vi "Main.vi"(11 "Module Admin":refnum<class "Delacor_lib_QMH_Module Admin.lvclass">) -> ()   [LabVIEW 2025, in "Power Supply.lvlib"]
doc: "This template is based from the Queued Message Handler design pattern and the Queued Message Handler Project Template that ships with LabVIEW 2014.\n\nThe main difference is that the Queue is private to this module and communication between modules is done via Broadcast and Request events.\n\nRequest events are wrapped via public API methods and are handled in the Event handler loop in this VI.\nAny module can register for Broadcast events sent by this module.\n\nThe Event Handling Loop generates messages based on user interface actions.\n\nThe Message Handling Loop processes messages generated by the Event Handling Loop, or by other messages. The messages are string values, so new messages can be added easily to the Message Cases case structure in the Message Handling Loop. Each message cluster can also provide an optional value for Message Data, which is a variant that can be converted to whatever message-specific data is required.\n_____\nBased on Delacor QMH Project Template 3.1.0.34.\n\n<b>Note:</b> This VI was modified by the <b>Validate DQMH Module</b> tool to add a call to the Error Reported VI at the end of the 'Exit' MHL frame.\n\n<b>Note:</b> This VI was modified by the <b>Validate DQMH Module</b> tool to call the Release Message Queue VI in the top-level Error case."
uses:
  Power Supply.lvlib
  <vilib>/Delacor/Delacor QMH/Libraries/Module Admin_class/Delacor_lib_QMH_Module Admin.lvclass
  <vilib>/MGI/Panel Manager/Panel/Panel/Panel.lvclass
  Module Data--cluster.ctl
  TV-STK-01/Plugins/PowerSupplies/PowerSupply/PowerSupply.lvlibp/PowerSupply/PowerSupply.lvclass
  Setpoints--cluster.ctl
  DC Output--enum.ctl
  Function Generator State--cluster.ctl
  Function Generator Parameters--cluster.ctl
  <vilib>/Utility/miscctls.llb/LVPointTypeDef.ctl
  <vilib>/Delacor/Delacor QMH/Libraries/Message Queue_class/Delacor_lib_QMH_Message Queue.lvclass/Delacor_lib_QMH_Message Queue.ctl
  Stop Argument--cluster.ctl
  <vilib>/Delacor/Delacor QMH/Libraries/Module Admin_class/Delacor_lib_QMH_Module Admin.lvclass/Delacor_lib_QMH_Module Admin.ctl
  Set Current SP Argument--cluster.ctl
  Set Voltage SP Argument--cluster.ctl
  Set Power SP Argument--cluster.ctl
  Set Power Supply Plugin Argument--cluster.ctl
  Set DC Output Argument--cluster.ctl
  Connect Argument--cluster.ctl
  Disconnect Argument--cluster.ctl
  Set Function Generator State Argument--cluster.ctl
  Set Function Generator Parameters Argument--cluster.ctl
  <vilib>/Delacor/Delacor QMH/Libraries/Message Queue_class/Delacor_lib_QMH_Enqueue Message (Single).vi
  <vilib>/Delacor/Delacor QMH/Libraries/Module Admin_class/Delacor_lib_QMH_Get External Launch.vi
  <vilib>/Utility/error.llb/Error Cluster From Error Code.vi
  <vilib>/ErrorRing/Error Ring.xnode
  <vilib>/Delacor/Delacor QMH/Libraries/Message Queue_class/Delacor_lib_QMH_Message Queue.lvclass
  <vilib>/MGI/Panel Manager/Panel/Panel Helper/Panel Helper.lvclass
  Get Status Argument--cluster.ctl
panel:
  out "Connected?":bool
  out "Function Generator State":T1
  out "Function Generator":T2
  out "Power Supply Status":T3
  out "Data Cluster":T4
  in  "Panel":refnum<class "Panel.lvclass">
  in  "Simulate MHL Error":bool
  in  "Simulate EHL Error":bool
  out "error out":errorcluster
  out "Status":string
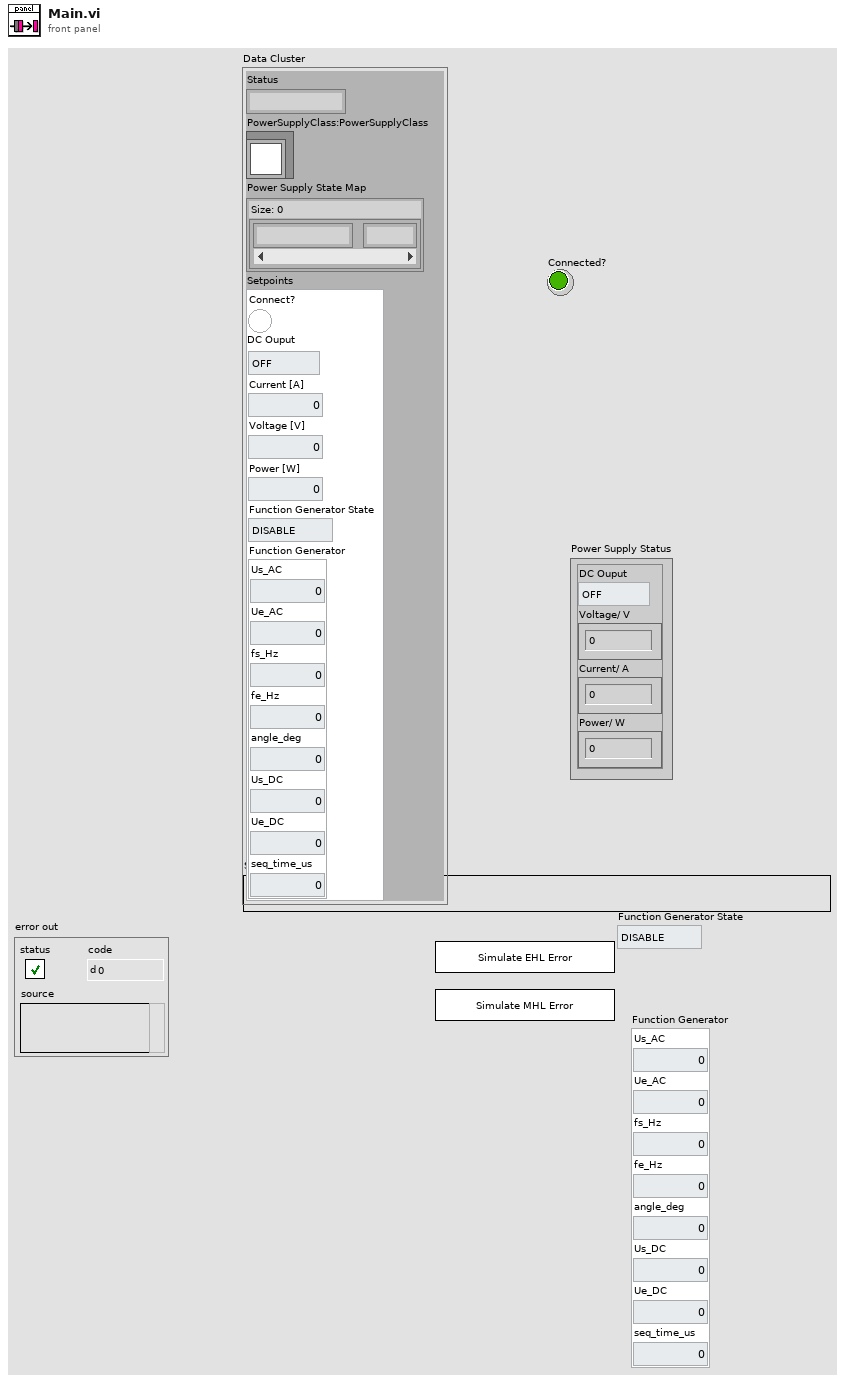
[diagram p1: front panel]
types:
  T1 = typedef "Power Supply.lvlib/Function Generator State--cluster.ctl" = enum16{"DISABLE", "ENABLE"}
  T2 = typedef "Power Supply.lvlib/Function Generator Parameters--cluster.ctl" = cluster{"Us_AC":sgl, "Ue_AC":sgl, "fs_Hz":sgl, "fe_Hz ":sgl, "angle_deg ":sgl, "Us_DC ":sgl, "Ue_DC":sgl, "seq_time_us":sgl}
  T3 = cluster{"DC Ouput":enum16{"OFF", "ON"}, "Voltage/ V":dbl, "Current/ A":dbl, "Power/ W":dbl}
  T4 = typedef "Power Supply.lvlib/Module Data--cluster.ctl" = cluster{"Status":string, "PowerSupplyClass:PowerSupplyClass":refnum<class "PowerSupply.lvclass">, "Power Supply State Map":map{string, dbl}, "Setpoints":T5}
  T5 = typedef "Power Supply.lvlib/Setpoints--cluster.ctl" = cluster{"Connect?":bool, "DC Ouput":T6, "Current [A]":dbl, "Voltage [V]":dbl, "Power [W]":dbl, "Function Generator State":T1, "Function Generator":T2}
  T6 = typedef "Power Supply.lvlib/DC Output--enum.ctl" = enum16{"OFF", "ON"}
  T7 = typedef "LVPointTypeDef.ctl" = cluster{"Horizontal":i16, "Vertical":i16}
  T8 = typedef "Power Supply.lvlib/Request Events--cluster.ctl" = cluster{"Stop Module":refnum<user-event>, "Show Panel":refnum<user-event>, "Hide Panel":refnum<user-event>, "Get Module Execution Status":refnum<user-event>, "Show Diagram":refnum<user-event>, "Change Panel":refnum<user-event>, "Set Current SP":refnum<user-event>, "Set Voltage SP":refnum<user-event>, "Set Power SP":refnum<user-event>, "Set Power Supply Plugin":refnum<user-event>, "Set DC Output":refnum<user-event>, "Private":cluster{"Sleep Connection Helper Loop":refnum<user-event>}, "Connect":refnum<user-event>, "Disconnect":refnum<user-event>, "Set Function Generator State":refnum<user-event>, "Private.Wake Connection Helper Loop":refnum<user-event>, "Private.Set DC Current SP":refnum<user-event>, "Private.Set DC Voltage SP":refnum<user-event>, "Private.Set DC Power SP":refnum<user-event>, "Private.Set DC Output SP":refnum<user-event>, "Set Function Generator Parameters":refnum<user-event>, "Private.Set Function Generator Parameters SP":refnum<user-event>, "Private.Set Function Generator State SP":refnum<user-event>}
  T9 = typedef "Panel.lvlib/Panel Helper.lvclass/Panel Events.ctl" = cluster{"My Panel":refnum<user-event>, "Top Level Initialized":refnum<user-event>}
  T10 = typedef "Power Supply.lvlib/Get Status Argument--cluster.ctl" = cluster{"Boolean":bool}
  T11 = typedef "Power Supply.lvlib/Stop Argument--cluster.ctl" = cluster{"Origin":string, "Exit via Stop Module Req?":bool, "Wait for Module to stop?":bool}
  T12 = typedef "Power Supply.lvlib/Set Current SP Argument--cluster.ctl" = cluster{"Current SP [A]":dbl}
  T13 = typedef "Power Supply.lvlib/Set Voltage SP Argument--cluster.ctl" = cluster{"Voltage SP [V]":dbl}
  T14 = typedef "Power Supply.lvlib/Set Power SP Argument--cluster.ctl" = cluster{"Power [W]":dbl}
  T15 = typedef "Power Supply.lvlib/Set Power Supply Plugin Argument--cluster.ctl" = cluster{"Plugin File Path":path}
  T16 = typedef "Power Supply.lvlib/Set DC Output Argument--cluster.ctl" = cluster{"DC Ouput":T6}
  T17 = typedef "Power Supply.lvlib/Connect Argument--cluster.ctl" = cluster{"Boolean":bool}
  T18 = typedef "Power Supply.lvlib/Disconnect Argument--cluster.ctl" = cluster{"Boolean":bool}
  T19 = typedef "Power Supply.lvlib/Set Function Generator State Argument--cluster.ctl" = cluster{"Function Generator State":T1}
  T20 = typedef "Power Supply.lvlib/Set Function Generator Parameters Argument--cluster.ctl" = cluster{"Function Generator":T2}
  T21 = enum32{"invalid lock state", "Not Locked", "Locked (No Password)", "Password-protected"}
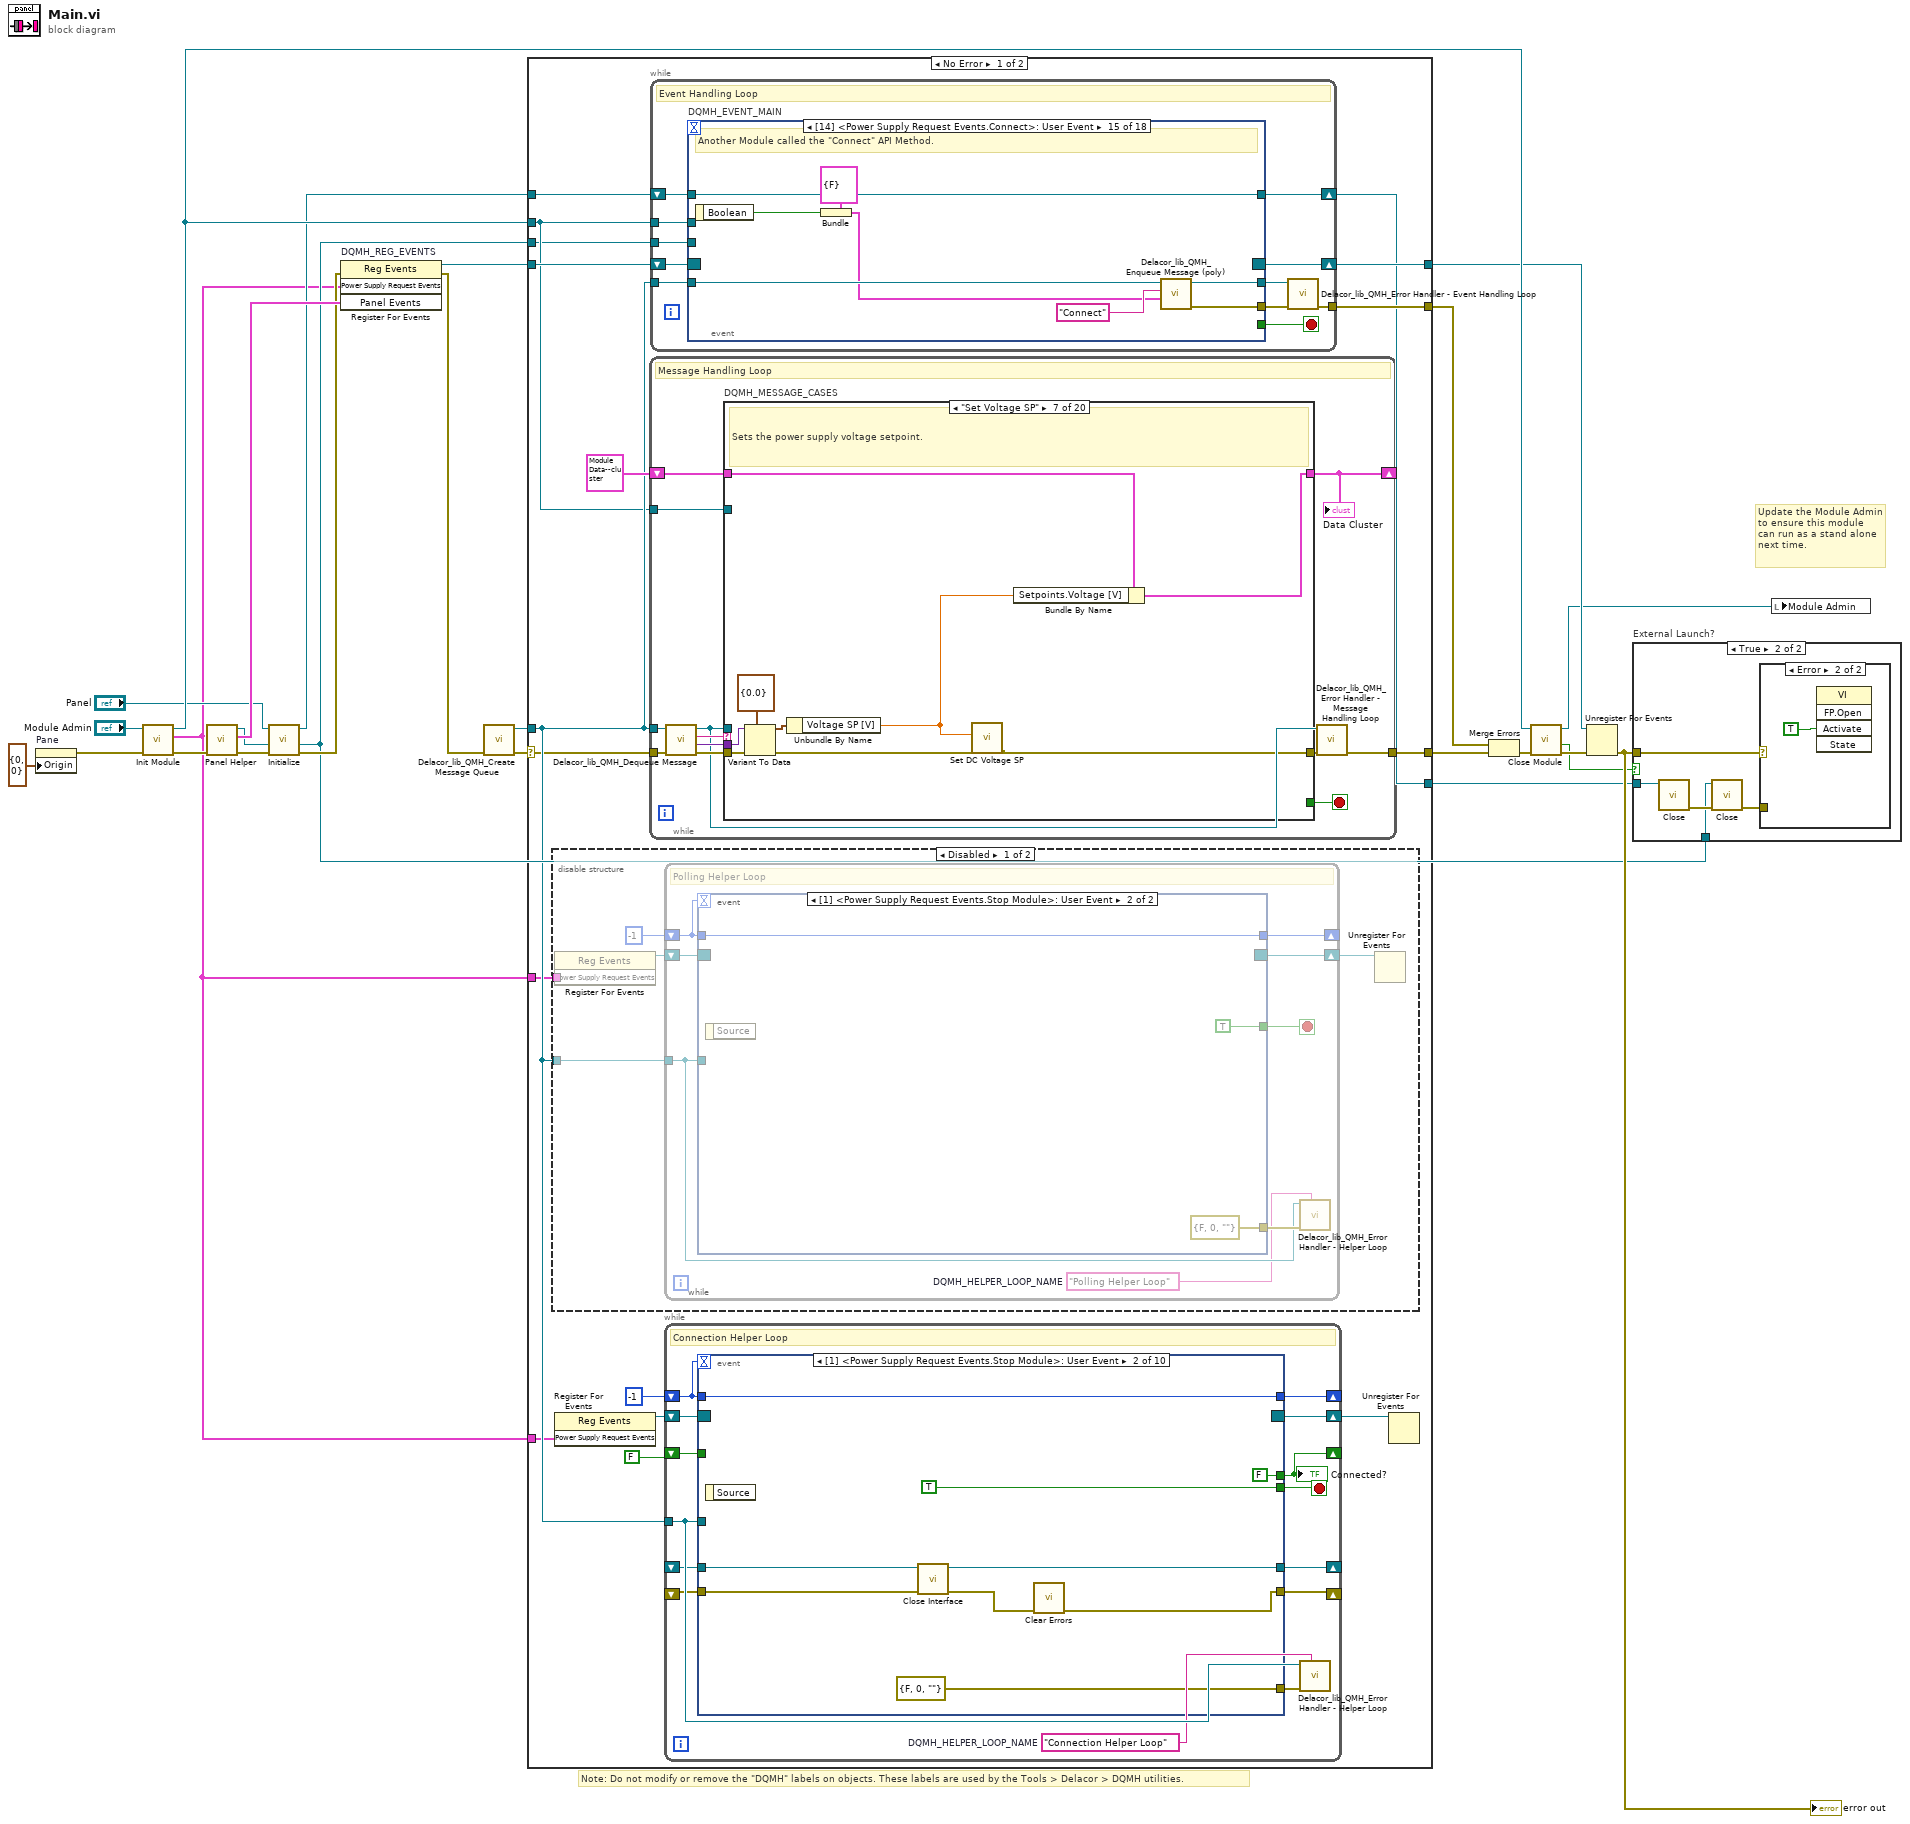
[diagram p0: block diagram]
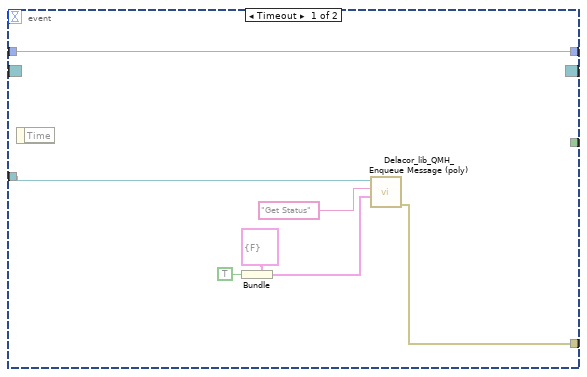
[diagram p4: hidden frame]
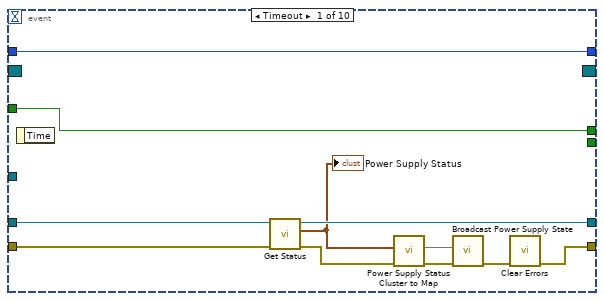
[diagram p6: hidden frame]
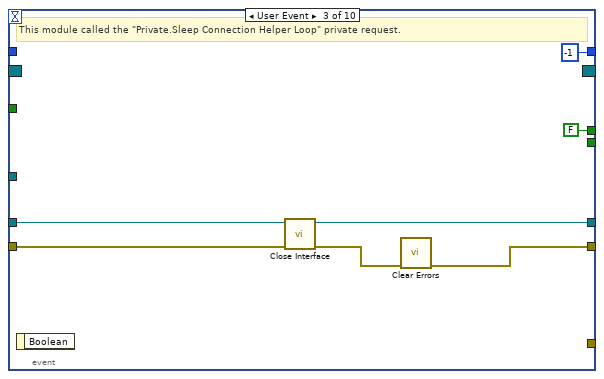
[diagram p7: hidden frame]
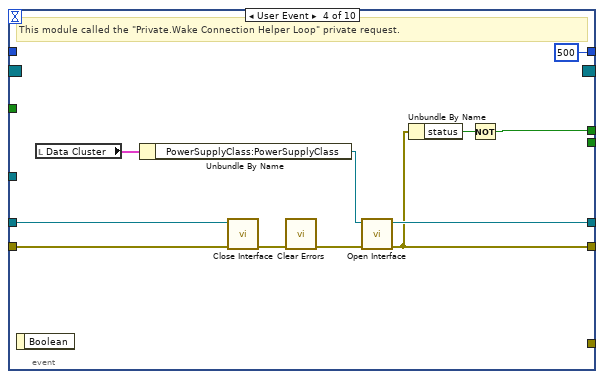
[diagram p8: hidden frame]
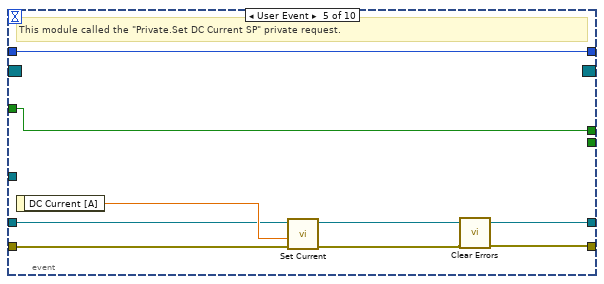
[diagram p9: hidden frame]
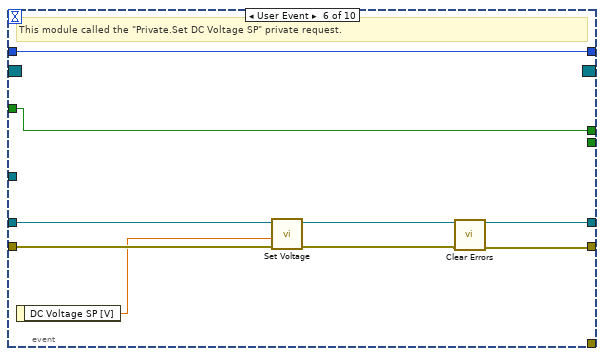
[diagram p10: hidden frame]
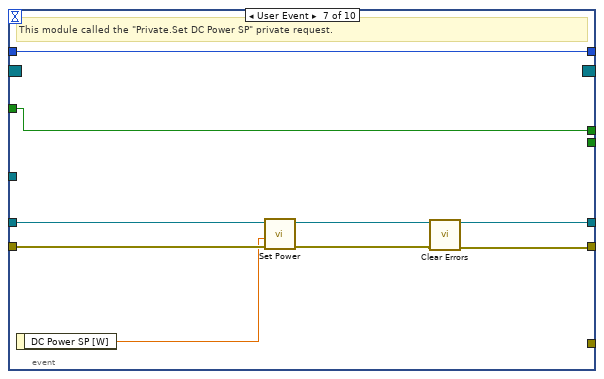
[diagram p11: hidden frame]
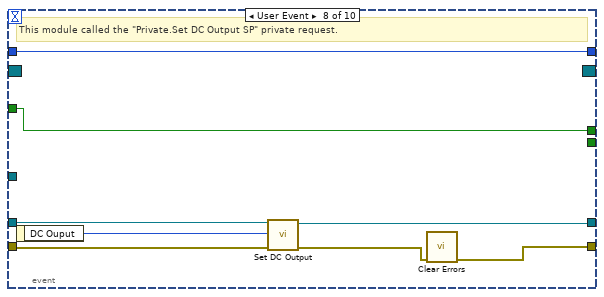
[diagram p12: hidden frame]
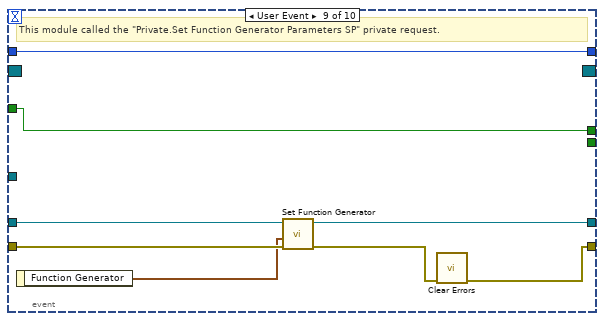
[diagram p13: hidden frame]
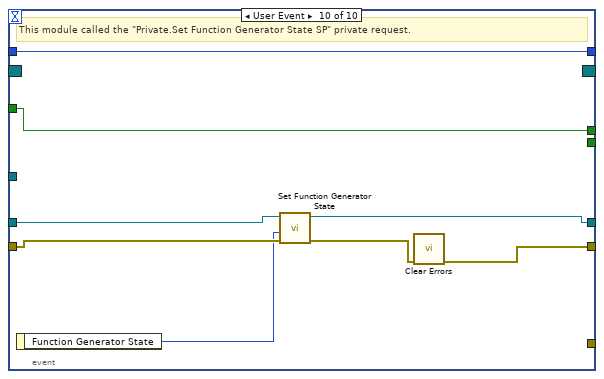
[diagram p14: hidden frame]
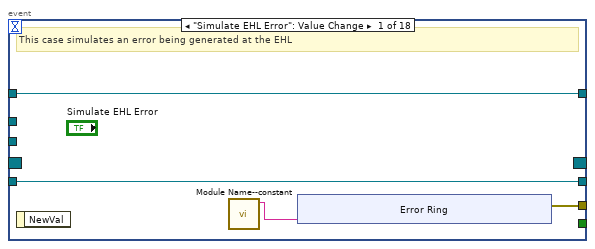
[diagram p15: hidden frame]
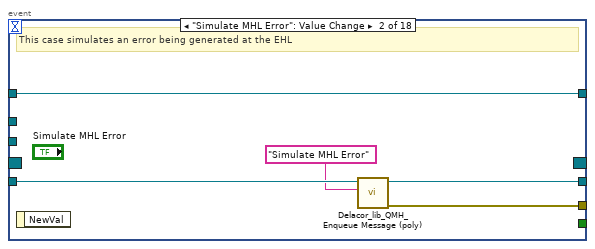
[diagram p16: hidden frame]
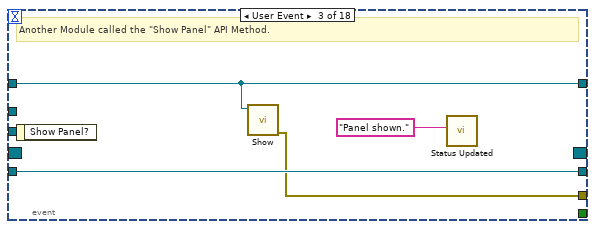
[diagram p17: hidden frame]
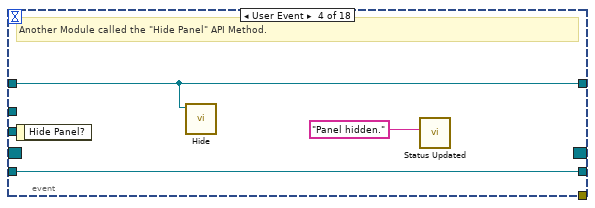
[diagram p18: hidden frame]
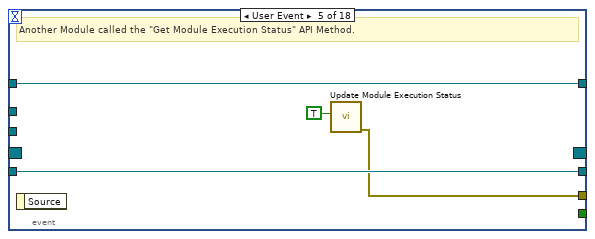
[diagram p19: hidden frame]
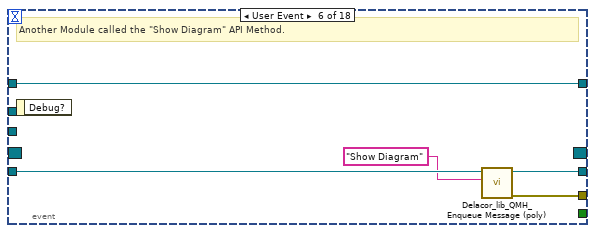
[diagram p20: hidden frame]
diagram:
  # "Note: Do not modify or remove the \"DQMH\" labels on objects. These labels are used by the Tools > Delacor > DQMH utilities."
  # "Update the Module Admin to ensure this module can run as a stand alone next time."
  n1 = property on="Pane" class="Pane"("Origin"=T7 {"Horizontal"=0, "Vertical"=0}) -> (error out=w2:errorcluster)  [unwired: 2 in, 1 out]
  n2 = call "Init Module.vi"("error in (no error)"=w2, "Singleton Module Admin in"="Module Admin") -> ("error out"=w12:errorcluster, "Power Supply Request Events"=w1:T8, "Singleton Module Admin out"=w26:refnum<class "Delacor_lib_QMH_Module Admin.lvclass">)  [unwired: 7 in]
  n3 = call <vilib>:"Panel Helper.vi"("Error In"=w12) -> ("Error Out"=w9:errorcluster, "Panel Events"=w11:T9, "Panel Helper out"=w8:refnum<class "Panel Helper.lvclass">)  [unwired: 8 in]
  n4 = call <vilib>:"Initialize.vi"("error in (no error)"=w9, "My Helper in"=w8, "Panel In"="Panel") -> ("error out"=w6:errorcluster, "My Helper out"=w5:refnum<class "Panel Helper.lvclass">, "Panel Out"=w4:refnum<class "Panel.lvclass">)  [unwired: 6 in]
  n5 = register-events "DQMH_REG_EVENTS"(error in=w6, w1, w11) -> (reference out=w23:refnum<event-registration>, error out=w10:errorcluster)  [unwired: 1 in]
  n6 = call <vilib>:"Delacor_lib_QMH_Create Message Queue.vi"("error in"=w10) -> ("error out"=w14:errorcluster, "Message Queue"=w22:refnum<class "Delacor_lib_QMH_Message Queue.lvclass">)  [unwired: 9 in]
  n7 = case shown="No Error" w14 {
    selector: w14 -> [w37 w520]
    tunnel: [w43 w520] -> w25
    tunnel: [w42 w525] -> w24
    tunnel: w23 -> [w40 w525]
    tunnel: w22 -> [w39 w516]
    tunnel: [w38 _] -> w18
    tunnel: w26 -> [w36 w521]
    tunnel: w4 -> [w34 w517]
    tunnel: w5 -> [w35 _]
    tunnel: [w33 w517] -> w13
    tunnel: w1 -> [w32 _]
    tunnel: w1 -> [w31 _]
    frame No Error {
      n8 = disable-structure shown="Disabled" {
        disable-tunnel: w39 -> [w48 _]
        disable-tunnel: w32 -> [w47 _]
        frame Disabled {
          n9 = register-events ("DQMH_HELPER_REGFOREVENTS")(w47) -> (reference out=w45:refnum<event-registration>)  [unwired: 2 in, 1 out]
          n10 = while "DQMH_HELPER_LOOP" {
            shift-right: [w56] -> _
            shift-left: -1 -> [w55]
            shift-right: [w53] -> w46
            shift-left: w45 -> [w54]
            tunnel: w48 -> [w50]
            stop <- w52 stop-if-true
            w49 = "Polling Helper Loop"  # DQMH_HELPER_LOOP_NAME
            # "Polling Helper Loop"
            n11 = event "DQMH_HELPER_EVENT_STRUCTURE" shown="[1] <Power Supply Request Events.Stop Module>: User Event" {
              selector: w54 -> [_ _]
              dyn-events: [_ _] -> w53
              timeout: w55 -> [_ _]
              tunnel: w55 -> [w63 w66]
              tunnel: [w63 w66] -> w56
              tunnel: [_ TRUE] -> w52
              tunnel: [w62 errorcluster {"status"=FALSE, "code"=0, "source"=""} ("error constant")] -> w51
              tunnel: w50 -> [w57 _]
              event Timeout {
                n12 = event-data() -> ()  [unwired: 1 in, 1 out]
                n13 = Bundle(cluster=T10 {"Boolean"=FALSE} ("Get Status Argument"), "Boolean"=TRUE) -> (w59:T10)
                n14 = call-poly <vilib>:"Delacor_lib_QMH_Enqueue Message (poly).vi"("Message Data"=w59, "Message"="Get Status", "Message Queue in"=w57) -> ("error out"=w62:errorcluster)  [unwired: 7 in, 1 out]
              }
              event User Event {
                n15 = event-data() -> ()  [unwired: 1 in, 1 out]
              }
            }
            n16 = call-dynamic "Delacor_lib_QMH_Error Handler - Helper Loop.vi"("Error Debug"=w49, "error in"=w51, "Message Queue in"=w50) -> ()  [unwired: 7 in, 2 out]
          }
          n17 = Unregister For Events(event registration refnum=w46) -> ()  [unwired: 1 in, 1 out]
        }
        frame Enabled {
        }
      }
      n18 = register-events ("DQMH_HELPER_REGFOREVENTS")(w31) -> (reference out=w29:refnum<event-registration>)  [unwired: 2 in, 1 out]
      n19 = while {
        tunnel: w39 -> [w323]
        shift-right: [w329] -> _
        shift-left: T4 {"Status"="", "PowerSupplyClass:PowerSupplyClass"=refnum, "Power Supply State Map"={}, "Setpoints"={"Connect?"=FALSE, "DC Ouput"=enum."OFF", "Current [A]"=0.0, "Voltage [V]"=0.0, "Power [W]"=0.0, "Function Generator State"=enum."DISABLE", "Function Generator"={"Us_AC"=0.0, "Ue_AC"=0.0, "fs_Hz"=0.0, "fe_Hz "=0.0, "angle_deg "=0.0, "Us_DC "=0.0, "Ue_DC"=0.0, "seq_time_us"=0.0}}} ("Data Cluster") -> [w330]
        tunnel: w37 -> [w327]
        tunnel: [w321] -> w43
        tunnel: w36 -> [w320]
        stop <- w328 stop-if-true
        # "Message Handling Loop"
        n20 = call-dynamic "Delacor_lib_QMH_Dequeue Message.vi"("error in"=w327, "Message Queue in"=w323) -> ("error out"=w326:errorcluster, "Message Data"=w324:variant, "Message"=w325:string, "Message Queue out"=w322:refnum<class "Delacor_lib_QMH_Message Queue.lvclass">)  [unwired: 6 in]
        n21 = case "DQMH_MESSAGE_CASES" shown="\"Set Voltage SP\"" w325 {
          selector: w325 -> [_ _ _ _ _ _ _ _ _ _ _ _ _ _ _ _ _ _ _ w505]
          tunnel: w322 -> [_ _ _ _ _ _ _ _ _ _ _ _ _ _ _ _ w468 w483 w501 _]
          tunnel: w326 -> [w334 w348 w352 w370 w376 w385 w394 w403 w412 w420 w428 w437 w446 w449 w452 w457 w474 w487 w503 _]
          tunnel: [w337 w349 w351 w368 w374 w380 w389 w398 w407 w416 w424 w432 w441 w447 w450 w455 w465 w485 w498 w506] -> w331
          tunnel: w330 -> [w342 w350 w353 w369 w375 w379 w388 w397 w405 w415 w422 w431 w440 w448 w451 w456 w473 w486 w489 w507]
          tunnel: [w341 w350 w353 w369 w375 w378 w387 w396 w404 w414 w421 w430 w439 w448 w451 w456 w473 w486 w489 w507] -> w329
          tunnel: [_ _ _ _ _ _ _ _ _ _ _ _ _ _ _ _ _ _ w500 _] -> w328
          tunnel: w324 -> [_ w347 _ _ w373 w384 w393 w402 w411 w419 w427 w436 w445 _ _ _ w472 _ w497 _]
          tunnel: w320 -> [w335 _ _ _ _ _ _ _ _ _ _ _ _ _ _ _ w467 _ w491 _]
          frame "Initialize" {
            w340 = "Initial Message" ("Initial Message")
            # "#CodeNeeded - Initialize your state data here."
            # "Initialize - Any operation that needs to be done before the module can receive messages. Synchronize Caller Events.vi will inform Start Module.vi that the module has launched and is ready to receive messages. Module Did Init.vi will broadcast that the module initialized."
            n22 = call "Create Power Supply.vi"("error in"=w334) -> ("error out"=w333:errorcluster, "Power Supply Interface out"=w332:refnum<class "PowerSupply.lvclass">)  [unwired: 9 in]
            n23 = call "Synchronize Caller Events.vi"("error in (no error)"=w333, "Singleton Module Admin in"=w335) -> ("error out"=w336:errorcluster)  [unwired: 8 in, 1 out]
            n24 = Bundle By Name(cluster=w342, "Status"=w340, "PowerSupplyClass:PowerSupplyClass"=w332) -> (w341:T4)
            n25 = call "Module Name--constant.vi"() -> ("Module Name"=w338:string)  [unwired: 11 in]
            n26 = local write "Status"(w340) -> ()
            n27 = call "Module Did Init.vi"("error in (no error)"=w336, "Initialized?"=TRUE, "Origin"=w338) -> ("error out"=w337:errorcluster)  [unwired: 8 in]
          }
          frame "Update Display" {
            # "Broadcast updated status to any VI registered to listen to this module's broadcast events."
            # "Convert the message data to a string to display in the Status indicator."
            # "#CodeRecommended - If you wish to decouple the Message Handling Loop from your user interface, consider creating User Events (like the \"Stop\" event in this VI) to message the Event Handling Loop whenever the user interface needs updating."
            # "Update Display - Update user interface here."
            n28 = Variant To Data(error in=w348, type="" ("Empty String Constant"), Variant=w347) -> (data=w345:string, error out=w344:errorcluster)
            "Status" <- w345
            n29 = call "Status Updated.vi"("error in (no error)"=w344, "Status"=w345) -> ("error out"=w343:errorcluster)  [unwired: 9 in]
            n30 = Merge Errors(w343) -> (w349:errorcluster)
          }
          frame "Show Diagram" {
            # "Show Diagram - Show the block diagram of this VI. Used as a debugging tool. There is a button in the module tester that fires the Show Diagram request, which runs this message. Note that the diagram will not be displayed if it is password-protected and the password is not in the cache."
            n31 = disable-structure shown="RUN_TIME_ENGINE==False" {
              disable-tunnel: [w361 w367] -> w351
              disable-tunnel: w352 -> [w360 w367]
              frame condition #0 (active) {
                # "functionality not available in exe"
                n32 = invoke on="Invoke Node" class="VI" method="Lock State.Get"(error in=w360) -> (error out=w359:errorcluster, "Get Lock State"=w358:T21, "pwd in cache"=w355:bool)  [unwired: 3 in, 1 out]
                n33 = Equal?(x=T21."Password-protected", y=w358) -> (x = y?=w356:bool)
                n34 = Compound Arithmetic op=AND(w356, invert w355) -> (w354:bool)
                n35 = case shown="False" w354 {
                  tunnel: [w364 w366] -> w361
                  tunnel: w359 -> [w362 w366]
                  frame False {
                    n36 = property on="Property Node" class="VI"(error in=w362, "BDWin.Open"=TRUE ("Block Diagram Window:Open")) -> (error out=w364:errorcluster)  [unwired: 1 in, 1 out]
                    n37 = call "Status Updated.vi"("Status"="Block Diagram shown." ("format string")) -> ()  [unwired: 10 in, 1 out]
                  }
                  frame True {
                    # "Password-protected VI, and the password is not in the cache. Do not show the diagram."
                  }
                }
              }
              frame condition #1 {
              }
            }
          }
          frame "--- Module Specific ---" {
            # "Separator -- The following cases handle messages specific to this Module."
            n38 = Merge Errors(w370) -> (w368:errorcluster)
          }
          frame "Set Power Supply Plugin" {
            # "Sets the power supply plugin path."
            n39 = Variant To Data(error in=w376, type=T15 {"Plugin File Path"=path ""} ("Set Power Supply Plugin Argument"), Variant=w373) -> (data=w371:T15, error out=w374:errorcluster)
            n40 = Unbundle By Name(w371) -> ()  [unwired: 1 out]
          }
          frame "Set Current SP" {
            # "Sets the power supply current setpoint."
            n41 = Variant To Data(error in=w385, type=T12 {"Current SP [A]"=0.0} ("Set Current SP Argument"), Variant=w384) -> (data=w382:T12, error out=w381:errorcluster)
            n42 = Unbundle By Name(w382) -> ("Current SP [A]"=w377:dbl)
            n43 = call "Set DC Current SP.vi"("error in"=w381, "DC Current [A]"=w377) -> ("error out"=w380:errorcluster)  [unwired: 9 in]
            n44 = Bundle By Name(cluster=w379, "Setpoints.Current [A]"=w377) -> (w378:T4)
          }
          frame "Set Voltage SP" {
            # "Sets the power supply voltage setpoint."
            n45 = Variant To Data(error in=w394, type=T13 {"Voltage SP [V]"=0.0} ("Set Voltage SP Argument"), Variant=w393) -> (data=w391:T13, error out=w390:errorcluster)
            n46 = Unbundle By Name(w391) -> ("Voltage SP [V]"=w386:dbl)
            n47 = call "Set DC Voltage SP.vi"("error in"=w390, "DC Voltage SP [V]"=w386) -> ("error out"=w389:errorcluster)  [unwired: 9 in]
            n48 = Bundle By Name(cluster=w388, "Setpoints.Voltage [V]"=w386) -> (w387:T4)
          }
          frame "Set Power SP" {
            # "Sets the power supply power setpoint."
            n49 = Variant To Data(error in=w403, type=T14 {"Power [W]"=0.0} ("Set Power SP Argument"), Variant=w402) -> (data=w400:T14, error out=w399:errorcluster)
            n50 = Unbundle By Name(w400) -> ("Power [W]"=w395:dbl)
            n51 = call "Set DC Power SP.vi"("error in"=w399, "DC Power SP [W]"=w395) -> ("error out"=w398:errorcluster)  [unwired: 9 in]
            n52 = Bundle By Name(cluster=w397, "Setpoints.Power [W]"=w395) -> (w396:T4)
          }
          frame "Set DC Output" {
            # "Sets the DC output of the power supply."
            n53 = Variant To Data(error in=w412, type=T16 {"DC Ouput"=enum."OFF"} ("Set DC Output Argument"), Variant=w411) -> (data=w409:T16, error out=w408:errorcluster)
            n54 = Unbundle By Name(w409) -> ("DC Ouput"=w406:T6)
            n55 = call "Set DC Output SP.vi"("error in"=w408, "DC Ouput"=w406) -> ("error out"=w407:errorcluster)  [unwired: 9 in]
            n56 = Bundle By Name(cluster=w405, "Setpoints.DC Ouput"=w406) -> (w404:T4)
          }
          frame "Connect" {
            # "Connect to the power supply."
            n57 = Variant To Data(error in=w420, type=T17 {"Boolean"=FALSE} ("Connect Argument"), Variant=w419) -> (error out=w417:errorcluster)  [unwired: 1 out]
            n58 = call "Wake Connection Helper Loop.vi"("error in"=w417) -> ("error out"=w416:errorcluster)  [unwired: 10 in]
            n59 = Bundle By Name(cluster=w415, "Setpoints.Connect?"=TRUE) -> (w414:T4)
          }
          frame "Disconnect" {
            # "Disconnect from Power Supply."
            n60 = Variant To Data(error in=w428, type=T18 {"Boolean"=FALSE} ("Disconnect Argument"), Variant=w427) -> (error out=w425:errorcluster)  [unwired: 1 out]
            n61 = Bundle By Name(cluster=w422, "Setpoints.Connect?"=FALSE) -> (w421:T4)
            n62 = call "Sleep Connection Helper Loop.vi"("error in"=w425) -> ("error out"=w424:errorcluster)  [unwired: 10 in]
          }
          frame "Set Function Generator State" {
            # "Sets the function generator state."
            n63 = Variant To Data(error in=w437, type=T19 {"Function Generator State"=enum."DISABLE"} ("Set Function Generator State Argument"), Variant=w436) -> (data=w434:T19, error out=w433:errorcluster)
            n64 = Unbundle By Name(w434) -> ("Function Generator State"=w429:T1)
            "Function Generator State" <- w429
            n65 = call "Set Function Generator State SP.vi"("error in"=w433, "Function Generator State"=w429) -> ("error out"=w432:errorcluster)  [unwired: 9 in]
            n66 = Bundle By Name(cluster=w431, "Setpoints.Function Generator State"=w429) -> (w430:T4)
          }
          frame "Set Function Generator Parameters" {
            # "Sets the function generator parameters."
            n67 = Variant To Data(error in=w446, type=T20 {"Function Generator"={"Us_AC"=0.0, "Ue_AC"=0.0, "fs_Hz"=0.0, "fe_Hz "=0.0, "angle_deg "=0.0, "Us_DC "=0.0, "Ue_DC"=0.0, "seq_time_us"=0.0}} ("Set Function Generator Parameters Argument"), Variant=w445) -> (data=w443:T20, error out=w442:errorcluster)
            n68 = Unbundle By Name(w443) -> ("Function Generator"=w438:T2)
            "Function Generator" <- w438
            n69 = call "Set Function Generator Parameters SP.vi"("error in"=w442, "Function Generator"=w438) -> ("error out"=w441:errorcluster)  [unwired: 9 in]
            n70 = Bundle By Name(cluster=w440, "Setpoints.Function Generator"=w438) -> (w439:T4)
          }
          frame "---Copy This Frame---" {
            # "Duplicate this frame when creating new messages.  Change this comment in the duplicated frame to describe this message."
            n71 = Merge Errors(w449) -> (w447:errorcluster)
          }
          frame "--- Exit and Error Handling---" {
            # "Separator - The following cases handle errors and exit messages."
            n72 = Merge Errors(w452) -> (w450:errorcluster)
          }
          frame "Simulate MHL Error" {
            # "Simulate an error occurring at the MHL"
            n73 = call "Module Name--constant.vi"() -> ("Module Name"=w454:string)  [unwired: 11 in]
            n74 = xnode "Error Ring"("parameter 0"=w454) -> ("error out"=w453:errorcluster)
            n75 = Merge Errors(w457, w453) -> (w455:errorcluster)
          }
          frame "Error" {
            # "Error - Check the error message data and respond accordingly. This message is sent by the \"Error Handler\" VIs at the end of each loop in this application."
            n76 = property on="Property Node" class="Module Admin"(reference=w467) -> ("Accessors:External Launch"=w466:bool)  [unwired: 1 in, 2 out]
            n77 = Variant To Data(error in=w474, type=errorcluster {"status"=FALSE, "code"=0, "source"=""} ("error constant"), Variant=w472) -> (data=w475:errorcluster, error out=w470:errorcluster)
            n78 = call "Error Reported.vi"("Error"=w475) -> ()  [unwired: 10 in, 1 out]
            n79 = case shown="True" w466 {
              tunnel: [w480 _] -> w469
              tunnel: w468 -> [w479 _]
              tunnel: w475 -> [w476 _]
              frame False {
                # "If the module is running standalone, then pop up an error dialog and call the \"Exit\" message."
                n80 = call <vilib>:"Simple Error Handler.vi"("error in (no error)"=w476) -> ()  [unwired: 4 in, 5 out]
                n81 = call-poly <vilib>:"Delacor_lib_QMH_Enqueue Message (poly).vi"("Priority Message? (F)"=TRUE, "Message"="Exit", "Message Queue in"=w479) -> ("error out"=w480:errorcluster)  [unwired: 7 in, 1 out]
              }
              frame True {
                # "If the module was launched externally, calling the Error Reported broadcast VI is the only action performed by the \"Error\" message. The module's caller can then process the error appropriately."
              }
            }
            n82 = Merge Errors(w470, w469) -> (w465:errorcluster)
            n83 = local write "error out"(w465) -> ()
          }
          frame "Confirm Quit" {
            # "#CodeNeeded - If you want to provide an \"Are you sure\" dialog (or some other notification) before the application exits, place that code here. This message is typically sent from a Panel Close? event."
            # "Confirm Quit - Message that can confirm whether or not the user wants to exit the application."
            n84 = call-poly <vilib>:"Delacor_lib_QMH_Enqueue Message (poly).vi"("Priority Message? (F)"=TRUE, "error in"=w487, "Message"="Exit", "Message Queue in"=w483) -> ("error out"=w484:errorcluster)  [unwired: 6 in, 1 out]
            n85 = Merge Errors(w484) -> (w485:errorcluster)
          }
          frame "Exit" {
            w495 = 91  # 91: not all Exit messages will have an argument
            w500 = TRUE  # Stop the VI
            # "Release the message queue reference"
            # "Exit - Exit the application."
            n86 = Variant To Data(error in=w503, type=T11 {"Origin"="", "Exit via Stop Module Req?"=FALSE, "Wait for Module to stop?"=FALSE} ("Stop Argument"), Variant=w497) -> (data=w493:T11, error out=w496:errorcluster)
            n87 = Unbundle By Name(w489) -> ("PowerSupplyClass:PowerSupplyClass"=w488:refnum<class "PowerSupply.lvclass">)
            n88 = call <vilib>:"Clear Errors.vi"("error in (no error)"=w496, "specific error code to clear (0: all)"=w495) -> ("error out"=w502:errorcluster)  [unwired: 4 in, 1 out]
            n89 = call-dynamic "Delacor_lib_QMH_Release Message Queue.vi"("error in"=w502, "Message Queue"=w501) -> ("error out"=w499:errorcluster)  [unwired: 9 in]
            n90 = call-dynamic "Close Interface.vi"("Power Supply in"=w488) -> ("error out"=w490:errorcluster)  [unwired: 9 in, 1 out]
            n91 = call "Handle Exit.vi"("Stop Argument"=w493, "Admin in"=w491) -> ("error out"=w492:errorcluster)  [unwired: 8 in, 1 out]
            n92 = Merge Errors(w490, w492, w499) -> (w498:errorcluster)
            n93 = call "Error Reported.vi"("Error"=w498) -> ()  [unwired: 10 in, 1 out]
          }
          frame Default {
            # "'Default' case only runs if there is a message that isn't defined in any of the other cases.  Output a programming error."
            n94 = call "Module Name--constant.vi"() -> ("Module Name"=w504:string)  [unwired: 11 in]
            n95 = xnode "Error Ring"("parameter 0"=w505, "parameter 1"=w504) -> ("error out"=w506:errorcluster)
          }
        }
        "Data Cluster" <- w329
        n96 = call-dynamic "Delacor_lib_QMH_Error Handler - Message Handling Loop.vi"("error in"=w331, "Message Queue in"=w322) -> ("dup error in"=w321:errorcluster)  [unwired: 8 in, 1 out]
      }
      n97 = while {
        tunnel: w39 -> [w177]
        shift-right: [w175] -> w42
        shift-left: w40 -> [w176]
        tunnel: [w171] -> w38
        tunnel: w36 -> [w170]
        tunnel: w35 -> [w169]
        shift-right: [w167] -> w33
        shift-left: w34 -> [w168]
        stop <- w173 stop-if-true
        # "Event Handling Loop"
        n98 = event "DQMH_EVENT_MAIN" shown="[14] <Power Supply Request Events.Connect>: User Event" {
          selector: w176 -> [_ _ _ _ _ _ _ _ _ _ _ _ _ _ _ _ _ _]
          dyn-events: [_ _ _ _ _ _ _ _ _ _ _ _ _ _ _ _ _ _] -> w175
          timeout: _ -> [_ _ _ _ _ _ _ _ _ _ _ _ _ _ _ _ _ _]
          tunnel: [_ _ _ _ _ _ TRUE ("Discard?") _ _ _ _ _ _ _ _ _ _ _] -> w173
          tunnel: w177 -> [w181 w193 w197 w200 w204 w209 w221 w231 w238 w255 w263 w271 w279 w287 w295 w303 w311 w319]
          tunnel: [w180 w190 w195 _ w203 w206 w215 w227 w237 w248 w256 w264 w272 w280 w288 w296 w304 w312] -> w174
          tunnel: [w181 w192 w197 w200 w204 w208 w220 w231 w236 w253 w261 w269 w277 w285 w293 w301 w309 w317] -> w172
          tunnel: w170 -> [_ _ _ _ _ _ _ _ w235 _ _ _ _ _ _ _ _ _]
          tunnel: w169 -> [_ _ _ _ _ _ _ w226 _ _ _ _ _ _ _ _ _ _]
          tunnel: w168 -> [w178 w189 w196 w199 w201 w205 w210 w230 w233 w254 w262 w270 w278 w286 w294 w302 w310 w318]
          tunnel: [w178 w189 w196 w199 w201 w205 w210 w225 w232 w254 w262 w270 w278 w286 w294 w302 w310 w318] -> w167
          event "Simulate EHL Error": Value Change {
            # "This case simulates an error being generated at the EHL"
            n99 = event-data() -> ()  [unwired: 1 in, 1 out]
            n100 = call "Module Name--constant.vi"() -> ("Module Name"=w179:string)  [unwired: 11 in]
            n101 = xnode "Error Ring"("parameter 0"=w179) -> ("error out"=w180:errorcluster)
          }
          event "Simulate MHL Error": Value Change {
            # "This case simulates an error being generated at the EHL"
            n102 = event-data() -> ()  [unwired: 1 in, 1 out]
            n103 = call-poly <vilib>:"Delacor_lib_QMH_Enqueue Message (poly).vi"("Message"="Simulate MHL Error", "Message Queue in"=w193) -> ("error out"=w190:errorcluster, "Message Queue out"=w192:refnum<class "Delacor_lib_QMH_Message Queue.lvclass">)  [unwired: 8 in]
          }
          event User Event {
            # "Another Module called the \"Show Panel\" API Method."
            n104 = event-data() -> ()  [unwired: 1 in, 1 out]
            n105 = call <vilib>:"Show.vi"("Panel in"=w196) -> ("Error Out"=w195:errorcluster)  [unwired: 10 in]
            n106 = call "Status Updated.vi"("Status"="Panel shown." ("format string")) -> ()  [unwired: 10 in, 1 out]
          }
          event User Event {
            # "Another Module called the \"Hide Panel\" API Method."
            n107 = event-data() -> ()  [unwired: 1 in, 1 out]
            n108 = call <vilib>:"Hide.vi"("Panel In"=w199) -> ()  [unwired: 10 in, 1 out]
            n109 = call "Status Updated.vi"("Status"="Panel hidden." ("format string")) -> ()  [unwired: 10 in, 1 out]
          }
          event User Event {
            # "Another Module called the \"Get Module Execution Status\" API Method."
            n110 = event-data() -> ()  [unwired: 1 in, 1 out]
            n111 = call "Update Module Execution Status.vi"("Running?"=TRUE) -> ("error out"=w203:errorcluster)  [unwired: 10 in]
          }
          event User Event {
            # "Another Module called the \"Show Diagram\" API Method."
            n112 = event-data() -> ()  [unwired: 1 in, 1 out]
            n113 = call-poly <vilib>:"Delacor_lib_QMH_Enqueue Message (poly).vi"("Message"="Show Diagram", "Message Queue in"=w209) -> ("error out"=w206:errorcluster, "Message Queue out"=w208:refnum<class "Delacor_lib_QMH_Message Queue.lvclass">)  [unwired: 8 in]
          }
          event User Event {
            # "The Stop Module Event can get fired from the Exit message in the MHL. The queue gets destroyed in that case. If the queue no longer exists, the Enqueue Exit as a priority message will return error 1. It is safe to ignore, because the module is already exiting."
            # "Another Module called the \"Stop Module\" API Method  or the Message Handling Loop below."
            n114 = event-data() -> ("Origin"=w219:string, "Exit via Stop Module Req?"=w213:bool, "Wait for Module to stop?"=w212:bool)  [unwired: 1 in]
            n115 = call <vilib>:"Hide.vi"("Panel In"=w210) -> ()  [unwired: 10 in, 1 out]
            n116 = local write "Status"(w219) -> ()
            n117 = Bundle By Name(cluster=T11 {"Origin"="", "Exit via Stop Module Req?"=FALSE, "Wait for Module to stop?"=FALSE} ("Stop Argument"), "Exit via Stop Module Req?"=w213, "Wait for Module to stop?"=w212) -> (w211:T11)
            n118 = call-poly <vilib>:"Delacor_lib_QMH_Enqueue Message (poly).vi"("Priority Message? (F)"=TRUE, "Message Data"=w211, "Message"="Exit", "Message Queue in"=w221) -> ("error out"=w216:errorcluster, "Message Queue out"=w220:refnum<class "Delacor_lib_QMH_Message Queue.lvclass">)  [unwired: 6 in]
            n119 = call <vilib>:"Clear Errors.vi"("error in (no error)"=w216, "specific error code to clear (0: all)"=1) -> ("error out"=w215:errorcluster)  [unwired: 4 in, 1 out]
          }
          event User Event {
            # "Another Module called the \"Change Panel\" API Method."
            n120 = event-data() -> ("New Panel"=w229:refnum<class "Panel.lvclass">)  [unwired: 1 in]
            n121 = call-dynamic <vilib>:"Close.vi"("Panel In"=w230) -> ("Error Out"=w228:errorcluster)  [unwired: 10 in]
            n122 = call <vilib>:"Initialize.vi"("error in (no error)"=w228, "My Helper in"=w226, "Panel In"=w229) -> ("error out"=w227:errorcluster, "Panel Out"=w225:refnum<class "Panel.lvclass">)  [unwired: 6 in, 1 out]
            n123 = call "Status Updated.vi"("Status"="Panel changed.") -> ()  [unwired: 10 in, 1 out]
          }
          event Panel Close? {
            w239 = TRUE  # Discard the event so the 'Confirm Quit' message has a chance to run.
            # "If launched externally, closing the panel doesn't quit the VI."
            # "Send the 'Confirm Quit' message if the user closes the panel of the VI."
            n124 = event-data() -> ()  [unwired: 1 in, 1 out]
            n125 = property on="Property Node" class="Module Admin"(reference=w235) -> ("Accessors:External Launch"=w234:bool)  [unwired: 1 in, 2 out]
            n126 = case shown="True" w234 {
              tunnel: w238 -> [w244 w247]
              tunnel: [w243 w245] -> w237
              tunnel: [w242 w247] -> w236
              tunnel: w233 -> [w240 w246]
              tunnel: [w240 w246] -> w232
              frame False {
                n127 = call-poly <vilib>:"Delacor_lib_QMH_Enqueue Message (poly).vi"("Message"="Confirm Quit", "Message Queue in"=w244) -> ("error out"=w243:errorcluster, "Message Queue out"=w242:refnum<class "Delacor_lib_QMH_Message Queue.lvclass">)  [unwired: 8 in]
              }
              frame True {
                n128 = call <vilib>:"Hide.vi"("Panel In"=w246) -> ("Error Out"=w245:errorcluster)  [unwired: 10 in]
              }
            }
            n129 = event-data ("Event Filter Node")("Discard?"=w239) -> ()  [unwired: 1 in, 1 out]
          }
          event User Event {
            # "Another Module called the \"Set Current SP\" API Method."
            n130 = event-data() -> ("Current SP [A]"=w249:dbl)  [unwired: 1 in]
            n131 = Bundle(cluster=T12 {"Current SP [A]"=0.0} ("Set Current SP Argument"), "Current SP [A]"=w249) -> (w250:T12)
            n132 = call-poly <vilib>:"Delacor_lib_QMH_Enqueue Message (poly).vi"("Message Data"=w250, "Message"="Set Current SP", "Message Queue in"=w255) -> ("error out"=w248:errorcluster, "Message Queue out"=w253:refnum<class "Delacor_lib_QMH_Message Queue.lvclass">)  [unwired: 7 in]
          }
          event User Event {
            # "Another Module called the \"Set Voltage SP\" API Method."
            n133 = event-data() -> ("Voltage SP [V]"=w257:dbl)  [unwired: 1 in]
            n134 = Bundle(cluster=T13 {"Voltage SP [V]"=0.0} ("Set Voltage SP Argument"), "Voltage SP [V]"=w257) -> (w258:T13)
            n135 = call-poly <vilib>:"Delacor_lib_QMH_Enqueue Message (poly).vi"("Message Data"=w258, "Message"="Set Voltage SP", "Message Queue in"=w263) -> ("error out"=w256:errorcluster, "Message Queue out"=w261:refnum<class "Delacor_lib_QMH_Message Queue.lvclass">)  [unwired: 7 in]
          }
          event User Event {
            # "Another Module called the \"Set Power SP\" API Method."
            n136 = event-data() -> ("Power [W]"=w265:dbl)  [unwired: 1 in]
            n137 = Bundle(cluster=T14 {"Power [W]"=0.0} ("Set Power SP Argument"), "Power [W]"=w265) -> (w266:T14)
            n138 = call-poly <vilib>:"Delacor_lib_QMH_Enqueue Message (poly).vi"("Message Data"=w266, "Message"="Set Power SP", "Message Queue in"=w271) -> ("error out"=w264:errorcluster, "Message Queue out"=w269:refnum<class "Delacor_lib_QMH_Message Queue.lvclass">)  [unwired: 7 in]
          }
          event User Event {
            # "Another Module called the \"Set Power Supply Plugin\" API Method."
            n139 = event-data() -> ("Plugin File Path"=w273:path)  [unwired: 1 in]
            n140 = Bundle(cluster=T15 {"Plugin File Path"=path ""} ("Set Power Supply Plugin Argument"), "Plugin File Path"=w273) -> (w274:T15)
            n141 = call-poly <vilib>:"Delacor_lib_QMH_Enqueue Message (poly).vi"("Message Data"=w274, "Message"="Set Power Supply Plugin", "Message Queue in"=w279) -> ("error out"=w272:errorcluster, "Message Queue out"=w277:refnum<class "Delacor_lib_QMH_Message Queue.lvclass">)  [unwired: 7 in]
          }
          event User Event {
            # "Another Module called the \"Set DC Output\" API Method."
            n142 = event-data() -> ("DC Ouput"=w281:T6)  [unwired: 1 in]
            n143 = Bundle(cluster=T16 {"DC Ouput"=enum."OFF"} ("Set DC Output Argument"), "DC Ouput"=w281) -> (w282:T16)
            n144 = call-poly <vilib>:"Delacor_lib_QMH_Enqueue Message (poly).vi"("Message Data"=w282, "Message"="Set DC Output", "Message Queue in"=w287) -> ("error out"=w280:errorcluster, "Message Queue out"=w285:refnum<class "Delacor_lib_QMH_Message Queue.lvclass">)  [unwired: 7 in]
          }
          event User Event {
            # "Another Module called the \"Connect\" API Method."
            n145 = event-data() -> ("Boolean"=w289:bool)  [unwired: 1 in]
            n146 = Bundle(cluster=T17 {"Boolean"=FALSE} ("Connect Argument"), "Boolean"=w289) -> (w290:T17)
            n147 = call-poly <vilib>:"Delacor_lib_QMH_Enqueue Message (poly).vi"("Message Data"=w290, "Message"="Connect", "Message Queue in"=w295) -> ("error out"=w288:errorcluster, "Message Queue out"=w293:refnum<class "Delacor_lib_QMH_Message Queue.lvclass">)  [unwired: 7 in]
          }
          event User Event {
            # "Another Module called the \"Disconnect\" API Method."
            n148 = event-data() -> ("Boolean"=w297:bool)  [unwired: 1 in]
            n149 = Bundle(cluster=T18 {"Boolean"=FALSE} ("Disconnect Argument"), "Boolean"=w297) -> (w298:T18)
            n150 = call-poly <vilib>:"Delacor_lib_QMH_Enqueue Message (poly).vi"("Message Data"=w298, "Message"="Disconnect", "Message Queue in"=w303) -> ("error out"=w296:errorcluster, "Message Queue out"=w301:refnum<class "Delacor_lib_QMH_Message Queue.lvclass">)  [unwired: 7 in]
          }
          event User Event {
            # "Another Module called the \"Set Function Generator State\" API Method."
            n151 = event-data() -> ("Function Generator State"=w305:T1)  [unwired: 1 in]
            n152 = Bundle(cluster=T19 {"Function Generator State"=enum."DISABLE"} ("Set Function Generator State Argument"), "Function Generator State"=w305) -> (w306:T19)
            n153 = call-poly <vilib>:"Delacor_lib_QMH_Enqueue Message (poly).vi"("Message Data"=w306, "Message"="Set Function Generator State", "Message Queue in"=w311) -> ("error out"=w304:errorcluster, "Message Queue out"=w309:refnum<class "Delacor_lib_QMH_Message Queue.lvclass">)  [unwired: 7 in]
          }
          event User Event {
            # "Another Module called the \"Set Function Generator Parameters\" API Method."
            n154 = event-data() -> ("Function Generator"=w313:T2)  [unwired: 1 in]
            n155 = Bundle(cluster=T20 {"Function Generator"={"Us_AC"=0.0, "Ue_AC"=0.0, "fs_Hz"=0.0, "fe_Hz "=0.0, "angle_deg "=0.0, "Us_DC "=0.0, "Ue_DC"=0.0, "seq_time_us"=0.0}} ("Set Function Generator Parameters Argument"), "Function Generator"=w313) -> (w314:T20)
            n156 = call-poly <vilib>:"Delacor_lib_QMH_Enqueue Message (poly).vi"("Message Data"=w314, "Message"="Set Function Generator Parameters", "Message Queue in"=w319) -> ("error out"=w312:errorcluster, "Message Queue out"=w317:refnum<class "Delacor_lib_QMH_Message Queue.lvclass">)  [unwired: 7 in]
          }
        }
        n157 = call-dynamic "Delacor_lib_QMH_Error Handler - Event Handling Loop.vi"("error in"=w174, "Message Queue in"=w172) -> ("dup error in"=w171:errorcluster)  [unwired: 8 in, 1 out]
      }
      n158 = while "DQMH_HELPER_LOOP" {
        shift-right: [w80] -> _
        shift-left: -1 -> [w79]
        shift-right: [w77] -> w30
        shift-left: w29 -> [w78]
        tunnel: w39 -> [w74]
        shift-right: [w72] -> _
        shift-left: _ -> [w71]
        shift-right: [w70] -> _
        shift-left: _ -> [w69]
        shift-right: [w68] -> _
        shift-left: FALSE ("status") -> [w67]
        stop <- w76 stop-if-true
        w73 = "Connection Helper Loop"  # DQMH_HELPER_LOOP_NAME
        # "Connection Helper Loop"
        n159 = event "DQMH_HELPER_EVENT_STRUCTURE" shown="[1] <Power Supply Request Events.Stop Module>: User Event" {
          selector: w78 -> [_ _ _ _ _ _ _ _ _ _]
          dyn-events: [_ _ _ _ _ _ _ _ _ _] -> w77
          timeout: w79 -> [_ _ _ _ _ _ _ _ _ _]
          tunnel: w79 -> [w84 w100 _ _ w126 w134 w142 w150 w158 w166]
          tunnel: [w84 w100 -1 500 w126 w134 w142 w150 w158 w166] -> w80
          tunnel: [_ TRUE _ _ _ _ _ _ _ _] -> w76
          tunnel: [_ errorcluster {"status"=FALSE, "code"=0, "source"=""} ("error constant") _ _ _ _ _ _ _ _] -> w75
          tunnel: w74 -> [_ _ _ _ _ _ _ _ _ _]
          tunnel: [w88 w96 w104 w114 w123 w130 w138 w148 w154 w162] -> w72
          tunnel: w71 -> [w90 w97 w106 w113 w124 w133 w141 w149 w157 w165]
          tunnel: [w81 w95 w103 w110 w119 w127 w135 w143 w151 w159] -> w70
          tunnel: w69 -> [w89 w94 w105 w112 w122 w132 w140 w146 w156 w164]
          tunnel: [w83 FALSE ("status") FALSE ("status") w108 w121 w129 w137 w145 w153 w161] -> w68
          tunnel: w67 -> [w83 _ _ _ w121 w129 w137 w145 w153 w161]
          event Timeout {
            n160 = event-data() -> ()  [unwired: 1 in, 1 out]
            n161 = call-dynamic "Get Status.vi"("error in (no error)"=w89, "Power Supply in"=w90) -> ("error out"=w86:errorcluster, "Power Supply Status"=w87:T3, "Power Supply out"=w88:refnum<class "PowerSupply.lvclass">)  [unwired: 7 in]
            "Power Supply Status" <- w87
            n162 = call "Power Supply Status Cluster to Map.vi"("error in (no error)"=w86, "Power Supply Status"=w87) -> ("error out"=w85:errorcluster, "Power Supply Status Map"=w91:map{string, dbl})  [unwired: 8 in]
            n163 = call "Broadcast Power Supply State.vi"("error in"=w85, "Power Supply State"=w91) -> ("error out"=w82:errorcluster)  [unwired: 9 in]
            n164 = call <vilib>:"Clear Errors.vi"("error in (no error)"=w82) -> ("error out"=w81:errorcluster)  [unwired: 5 in, 1 out]
          }
          event User Event {
            n165 = event-data() -> ()  [unwired: 1 in, 1 out]
            n166 = call-dynamic "Close Interface.vi"("error in (no error)"=w94, "Power Supply in"=w97) -> ("error out"=w93:errorcluster, "Power Supply out"=w96:refnum<class "PowerSupply.lvclass">)  [unwired: 8 in]
            n167 = call <vilib>:"Clear Errors.vi"("error in (no error)"=w93) -> ("error out"=w95:errorcluster)  [unwired: 5 in, 1 out]
          }
          event User Event {
            # "This module called the \"Private.Sleep Connection Helper Loop\" private request."
            n168 = event-data() -> ()  [unwired: 1 in, 1 out]
            n169 = call-dynamic "Close Interface.vi"("error in (no error)"=w105, "Power Supply in"=w106) -> ("error out"=w102:errorcluster, "Power Supply out"=w104:refnum<class "PowerSupply.lvclass">)  [unwired: 8 in]
            n170 = call <vilib>:"Clear Errors.vi"("error in (no error)"=w102) -> ("error out"=w103:errorcluster)  [unwired: 5 in, 1 out]
          }
          event User Event {
            # "This module called the \"Private.Wake Connection Helper Loop\" private request."
            n171 = event-data() -> ()  [unwired: 1 in, 1 out]
            n172 = local read "Data Cluster"() -> (w115:T4)
            n173 = Unbundle By Name(w115) -> ("PowerSupplyClass:PowerSupplyClass"=w116:refnum<class "PowerSupply.lvclass">)
            n174 = call-dynamic "Close Interface.vi"("error in (no error)"=w112, "Power Supply in"=w113) -> ("error out"=w118:errorcluster)  [unwired: 8 in, 1 out]
            n175 = call <vilib>:"Clear Errors.vi"("error in (no error)"=w118) -> ("error out"=w117:errorcluster)  [unwired: 5 in, 1 out]
            n176 = call-dynamic "Open Interface.vi"("error in (no error)"=w117, "Power Supply in"=w116) -> ("error out"=w110:errorcluster, "Power Supply out"=w114:refnum<class "PowerSupply.lvclass">)  [unwired: 8 in]
            n177 = Unbundle By Name(w110) -> ("status"=w109:bool)
            n178 = Not(x=w109) -> (.not. x?=w108:bool)
          }
          event User Event {
            # "This module called the \"Private.Set DC Current SP\" private request."
            n179 = event-data() -> ("DC Current [A]"=w125:dbl)  [unwired: 1 in]
            n180 = call-dynamic "Set Current.vi"("error in (no error)"=w122, "Current/ A"=w125, "Power Supply in"=w124) -> ("error out"=w120:errorcluster, "Power Supply out"=w123:refnum<class "PowerSupply.lvclass">)  [unwired: 7 in]
            n181 = call <vilib>:"Clear Errors.vi"("error in (no error)"=w120) -> ("error out"=w119:errorcluster)  [unwired: 5 in, 1 out]
          }
          event User Event {
            # "This module called the \"Private.Set DC Voltage SP\" private request."
            n182 = event-data() -> ("DC Voltage SP [V]"=w131:dbl)  [unwired: 1 in]
            n183 = call-dynamic "Set Voltage.vi"("error in (no error)"=w132, "Voltage SP/ V"=w131, "Power Supply in"=w133) -> ("error out"=w128:errorcluster, "Power Supply out"=w130:refnum<class "PowerSupply.lvclass">)  [unwired: 7 in]
            n184 = call <vilib>:"Clear Errors.vi"("error in (no error)"=w128) -> ("error out"=w127:errorcluster)  [unwired: 5 in, 1 out]
          }
          event User Event {
            # "This module called the \"Private.Set DC Power SP\" private request."
            n185 = event-data() -> ("DC Power SP [W]"=w139:dbl)  [unwired: 1 in]
            n186 = call-dynamic "Set Power.vi"("error in (no error)"=w140, "Power SP/ W"=w139, "Power Supply in"=w141) -> ("error out"=w136:errorcluster, "Power Supply out"=w138:refnum<class "PowerSupply.lvclass">)  [unwired: 7 in]
            n187 = call <vilib>:"Clear Errors.vi"("error in (no error)"=w136) -> ("error out"=w135:errorcluster)  [unwired: 5 in, 1 out]
          }
          event User Event {
            # "This module called the \"Private.Set DC Output SP\" private request."
            n188 = event-data() -> ("DC Ouput"=w147:T6)  [unwired: 1 in]
            n189 = call-dynamic "Set DC Output.vi"("error in (no error)"=w146, "DC Output"=w147, "Power Supply in"=w149) -> ("error out"=w144:errorcluster, "Power Supply out"=w148:refnum<class "PowerSupply.lvclass">)  [unwired: 7 in]
            n190 = call <vilib>:"Clear Errors.vi"("error in (no error)"=w144) -> ("error out"=w143:errorcluster)  [unwired: 5 in, 1 out]
          }
          event User Event {
            # "This module called the \"Private.Set Function Generator Parameters SP\" private request."
            n191 = event-data() -> ("Function Generator"=w155:T2)  [unwired: 1 in]
            n192 = call-dynamic "Set Function Generator.vi"("error in (no error)"=w156, "Function Generator"=w155, "PowerSupplyClass in"=w157) -> ("error out"=w152:errorcluster, "PowerSupplyClass out"=w154:refnum<class "PowerSupply.lvclass">)  [unwired: 7 in]
            n193 = call <vilib>:"Clear Errors.vi"("error in (no error)"=w152) -> ("error out"=w151:errorcluster)  [unwired: 5 in, 1 out]
          }
          event User Event {
            # "This module called the \"Private.Set Function Generator State SP\" private request."
            n194 = event-data() -> ("Function Generator State"=w163:T1)  [unwired: 1 in]
            n195 = call-dynamic "Set Function Generator State.vi"("error in (no error)"=w164, "Function Generator State"=w163, "PowerSupplyClass in"=w165) -> ("error out"=w160:errorcluster, "PowerSupplyClass out"=w162:refnum<class "PowerSupply.lvclass">)  [unwired: 7 in]
            n196 = call <vilib>:"Clear Errors.vi"("error in (no error)"=w160) -> ("error out"=w159:errorcluster)  [unwired: 5 in, 1 out]
          }
        }
        "Connected?" <- w68
        n197 = call-dynamic "Delacor_lib_QMH_Error Handler - Helper Loop.vi"("Error Debug"=w73, "error in"=w75, "Message Queue in"=w74) -> ()  [unwired: 7 in, 2 out]
      }
      n198 = Unregister For Events(event registration refnum=w30) -> ()  [unwired: 1 in, 1 out]
    }
    frame Error {
      # "Synchronize Caller Events.vi will inform Start Module.vi that the module has launched and will let the code calling Start Module.vi register for broadcasts and would permit the caller receive the broadcast that an error occurred at launch time."
      n199 = call-dynamic "Delacor_lib_QMH_Release Message Queue.vi"("Message Queue"=w516) -> ()  [unwired: 10 in, 1 out]
      n200 = call "Synchronize Caller Events.vi"("Singleton Module Admin in"=w521) -> ("error out"=w518:errorcluster)  [unwired: 9 in, 1 out]
      n201 = call "Module Name--constant.vi"() -> ("Module Name"=w524:string)  [unwired: 11 in]
      n202 = Format Into String(format string="An error occurred during initialization. %s is no longer running.", w524) -> (resulting string=w522:string)  [unwired: 2 in, 1 out]
      n203 = Merge Errors(w520, w518) -> (w519:errorcluster)
      n204 = call "Error Reported.vi"("Additional Information"=w522, "Error"=w519) -> ()  [unwired: 9 in, 1 out]
    }
  }
  n205 = Merge Errors(w18, w25) -> (w17:errorcluster)
  n206 = call "Close Module.vi"("error in (no error)"=w17, "Module Admin in"=w26) -> ("error out"=w20:errorcluster, "External Launch"=w15:bool, "Module Admin out"=w19:refnum<class "Delacor_lib_QMH_Module Admin.lvclass">)  [unwired: 7 in]
  n207 = Unregister For Events(event registration refnum=w24, error in=w20) -> (error out=w16:errorcluster)
  "error out" <- w16
  n208 = case "External Launch?" shown="True" w15 {
    tunnel: w16 -> [_ w530]
    tunnel: w13 -> [_ w529]
    tunnel: w5 -> [_ w527]
    frame False {
    }
    frame True {
      n209 = call-dynamic <vilib>:"Close.vi"("Panel In"=w529) -> ("Error Out"=w528:errorcluster)  [unwired: 10 in]
      n210 = call <vilib>:"Close.vi"("error in (no error)"=w528, "Controller in"=w527) -> ("error out"=w526:errorcluster)  [unwired: 9 in]
      n211 = case shown="Error" w530 {
        tunnel: w526 -> [_ _]
        frame No Error {
        }
        frame Error {
          n212 = invoke on="Invoke Node" class="VI" method="FP.Open"("Activate"=TRUE ("Activate?")) -> ()  [unwired: 4 in, 5 out]
        }
      }
    }
  }
  n213 = local write "Module Admin"(w19) -> ()
